vi "SubVI2.vi"() -> ()   [LabVIEW 2021]
panel:
  in  "Close Button":bool
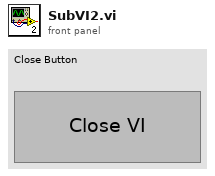
[diagram p1: front panel]
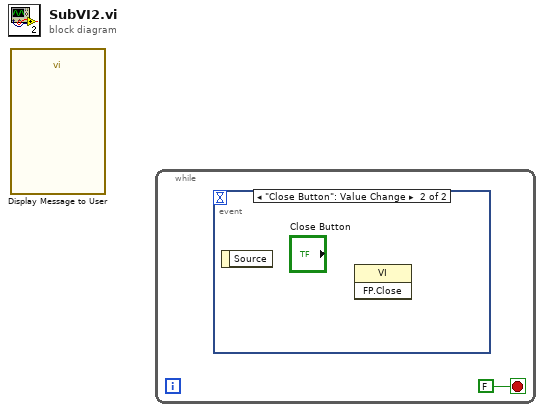
[diagram p0: block diagram]
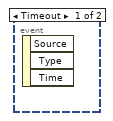
[diagram p2: hidden frame]
diagram:
  n1 = call "Display Message to User"() -> ()  [unwired: 10 in, 2 out]
  n2 = while {
    stop <- FALSE stop-if-true
    n3 = event shown="[1] \"Close Button\": Value Change" {
      selector: _ -> [_ _]
      dyn-events: _ -> [_ _]
      timeout: _ -> [_ _]
      event Timeout {
        n4 = event-data() -> ()  [unwired: 1 in, 3 out]
      }
      event "Close Button": Value Change {
        n5 = event-data() -> ()  [unwired: 1 in, 1 out]
        n6 = invoke class="VI" method="FP.Close"() -> ()  [unwired: 3 in, 3 out]
      }
    }
  }
